vi "Read I32.vi"(8 "error in (no error)":errorcluster, 11 "Event in":refnum<class "Event I32.lvclass">) -> (0 "error out":errorcluster, 2 "I32":i32, 3 "Event out":refnum<class "Event I32.lvclass">)   [LabVIEW 2017, in "Event Actors.lvlib" / "Event I32.lvclass"]
uses:
  Event I32.lvclass
  Event I32.lvclass/Event I32.ctl
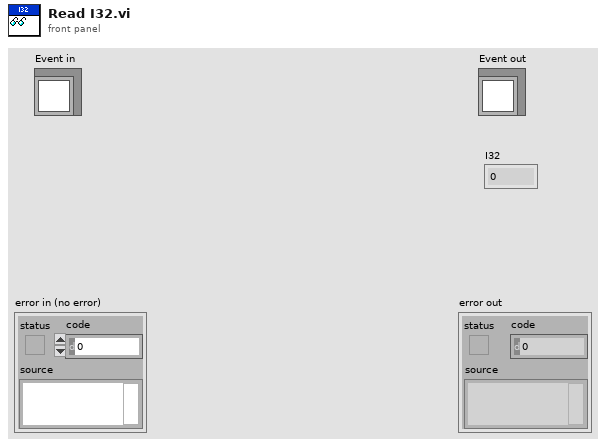
[diagram p1: front panel]
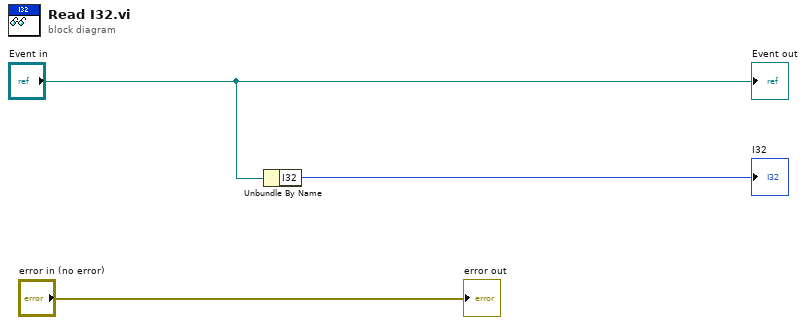
[diagram p0: block diagram]
diagram:
  n1 = Unbundle By Name("Event in") -> ("I32"=→"I32":i32)
  "Event out" <- "Event in"
  "error out" <- "error in (no error)"
